vi "二值化(子VI).vi"(11 "Manual":cluster{sgl, sgl}(slide)={0.0, 150.0} caption="Threshold Range" scale=0.0..255.0) -> (3 "引用句柄输出":T1(plugin-control))   [LabVIEW 2014]
uses:
  <vilib>/vision/NI_Vision_Development_Module.lvlib
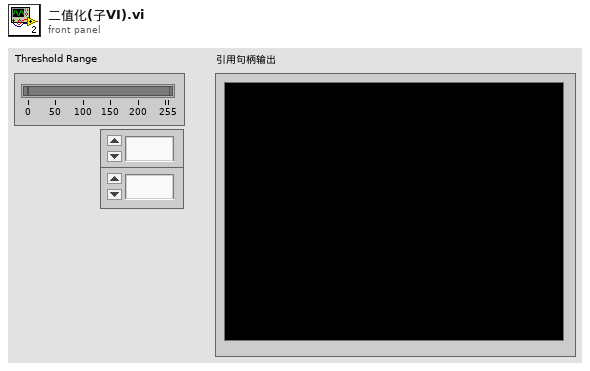
[diagram p1: front panel]
types:
  T1 = typedef "IMAQ Image.ctl" = refnum<image>
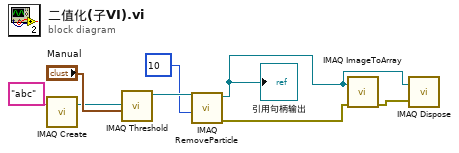
[diagram p0: block diagram]
diagram:
  n1 = call "IMAQ Create"("Image Name"="abc") -> ("New Image"=w4:T1)  [unwired: 4 in, 1 out]
  n2 = call "IMAQ Threshold"("Range"="Manual", "Image Dst"=w4) -> ("Image Dst Out"=w5:T1)  [unwired: 8 in, 1 out]
  n3 = call "IMAQ RemoveParticle"("Number of Erosion"=10, "Image Src"=w5) -> ("error out"=w3:errorcluster, "Image Dst Out"=w8:T1)  [unwired: 8 in]
  "引用句柄输出" <- w8
  n4 = call "IMAQ ImageToArray"("error in (no error)"=w3, "Image"=w8) -> ("error out"=w7:errorcluster)  [unwired: 2 in, 4 out]
  n5 = call "IMAQ Dispose"("Image"=w8, "error in (no error)"=w7) -> ()  [unwired: 4 in, 1 out]
